vi "Page_Source_Initialize.vi"(8 "error in (no error)":errorcluster, 9 "ctlReferences":T3, 11 "AB_SourceDistribution in":refnum<class "AB_SourceDistribution.lvclass">) -> (0 "error out":errorcluster, 1 "supportedFunctions":T1, 3 "AB_SourceDistribution out":refnum<class "AB_SourceDistribution.lvclass">)   [LabVIEW 2020, in "AB_SourceDistribution.lvclass"]
uses:
  <vilib>/AppBuilder/AB_Classes/SourceDistribution/AB_SourceDistribution.lvclass
  <resource>/Framework/Providers/Builds/AppBuilder/AB_UI_Page_Source_Files_References.ctl
  <resource>/Framework/Providers/Builds/AppBuilder/AB_UI_Page_Source_Files_supportedFunctions.ctl
  <vilib>/AppBuilder/AB_Source_Inclusion.ctl
  <resource>/Framework/Providers/Common/provcom_StringGlobals.vi
  <vilib>/AppBuilder/AB_Classes/Build/AB_Build.lvclass
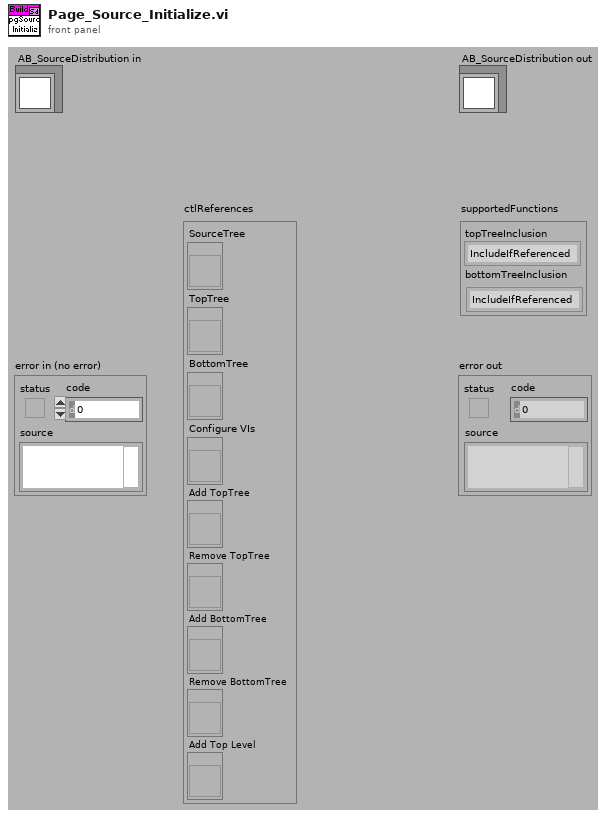
[diagram p1: front panel]
types:
  T1 = typedef "AB_UI_Page_Source_Files_supportedFunctions.ctl" = cluster{"topTreeInclusion":T2, "bottomTreeInclusion":T2}
  T2 = typedef "AB_Source_Inclusion.ctl" = enum16{"IncludeIfReferenced", "Include", "Exclude", "TopLevel"}
  T3 = typedef "AB_UI_Page_Source_Files_References.ctl" = cluster{"SourceTree":refnum<vi>, "TopTree":refnum<vi>, "BottomTree":refnum<vi>, "Configure VIs":refnum<vi>, "Add TopTree":refnum<vi>, "Remove TopTree":refnum<vi>, "Add BottomTree":refnum<vi>, "Remove BottomTree":refnum<vi>, "Add Top Level":refnum<vi>}
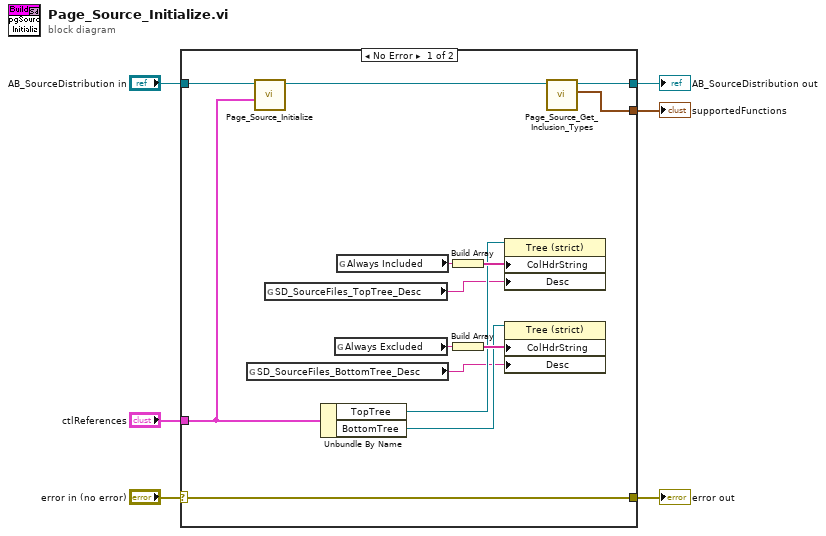
[diagram p0: block diagram]
diagram:
  n1 = case shown="No Error" "error in (no error)" {
    selector: "error in (no error)" -> [w14 w22]
    tunnel: [w14 w22] -> w5
    tunnel: [w11 w21] -> w3
    tunnel: "AB_SourceDistribution in" -> [w9 w21]
    tunnel: "ctlReferences" -> [w7 _]
    tunnel: [w10 _] -> w1
    frame No Error {
      n2 = global read "provcom_StringGlobals.vi" "SD_SourceFiles_BottomTree_Desc"() -> (w12:string)
      n3 = call-parent "Page_Source_Initialize.vi"("ctlReferences"=w7, "AB_Build in"=w9) -> ("AB_Build out"=w8:refnum<class "AB_SourceDistribution.lvclass">)  [unwired: 7 in, 2 out]
      n4 = global read "provcom_StringGlobals.vi" "SD_SourceFiles_TopTree_Desc"() -> (w13:string)
      n5 = Unbundle By Name(w7) -> ("TopTree"=w15:refnum<vi>, "BottomTree"=w16:refnum<vi>)
      n6 = global read "provcom_StringGlobals.vi" "Always Excluded"() -> (w17:string)
      n7 = global read "provcom_StringGlobals.vi" "Always Included"() -> (w20:string)
      n8 = Build Array(w20) -> (w19:string[])
      n9 = Build Array(w17) -> (w18:string[])
      n10 = property class="Tree (strict)"(reference=w15, "ColHdrString"=w19, "Desc"=w13) -> ()  [unwired: 1 in, 2 out]
      n11 = property class="Tree (strict)"(reference=w16, "ColHdrString"=w18, "Desc"=w12) -> ()  [unwired: 1 in, 2 out]
      n12 = call-dynamic "Page_Source_Get_Inclusion_Types.vi"("AB_SourceDistribution in"=w8) -> ("supportedFunctions"=w10:T1, "AB_SourceDistribution out"=w11:refnum<class "AB_SourceDistribution.lvclass">)  [unwired: 8 in, 1 out]
    }
    frame Error {
    }
  }
  "error out" <- w5
  "AB_SourceDistribution out" <- w3
  "supportedFunctions" <- w1
